vi "2. HelloWorld.vi"() -> ()   [LabVIEW 2019]
panel:
  out "String":string
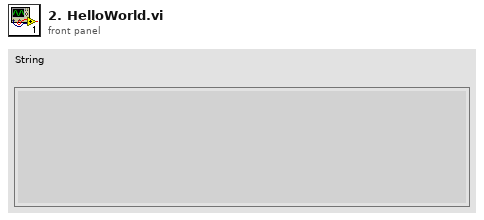
[diagram p1: front panel]
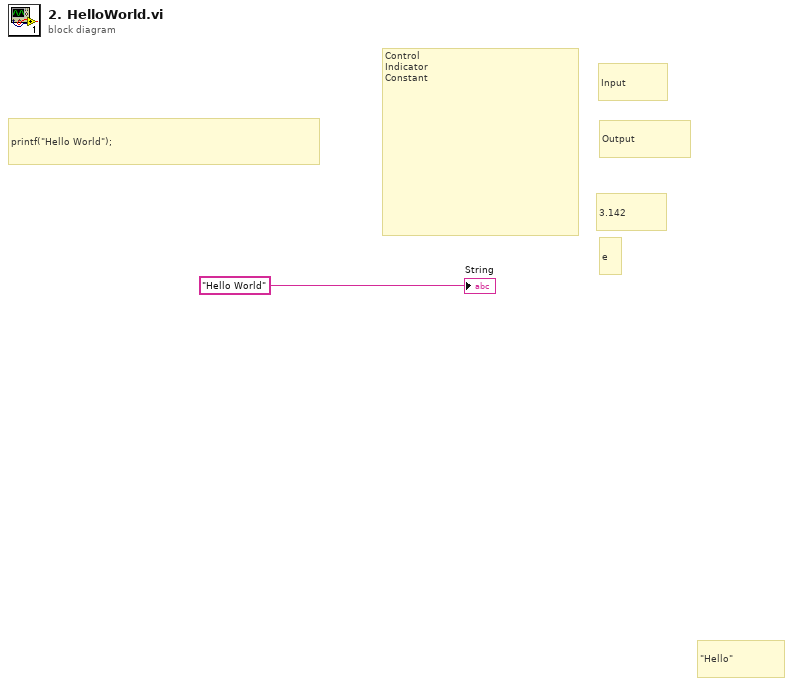
[diagram p0: block diagram]
diagram:
  # "printf(\"Hello World\");"
  # "\"Hello\""
  # "e"
  # "3.142"
  # "Output"
  # "Input"
  # "Control\nIndicator\nConstant"
  "String" <- "Hello World"
